vi "count from data base_0.vi"() -> ()   [LabVIEW 2015]
panel:
  in  "Tab Control":enum32{"Page 1", "Page 2"}(tab)
  out "Array":dbl[](array[numeric])
  in  "?":dbl
  out "Result":i16
  # "Count from data base"
  # "User enter value__ count in result how much int value greater than user enput"
  # "Pardeep Kumar"
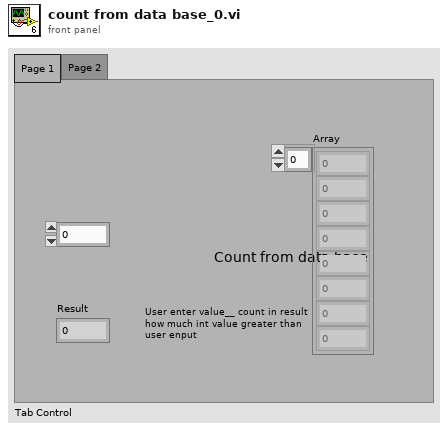
[diagram p1: front panel]
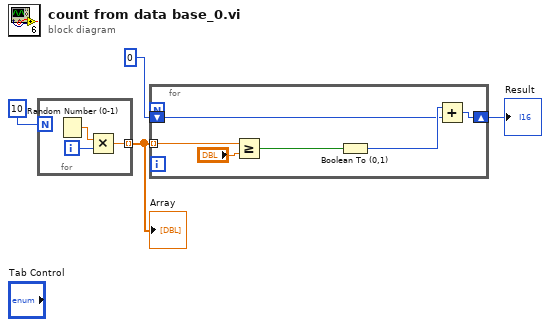
[diagram p0: block diagram]
diagram:
  n1 = for {
    N: 10 -> [_]
    tunnel: [w5] -> w3 mode=indexing
    i -> [w6]
    n2 = Random Number (0-1)() -> (number: 0 to 1=w7:dbl)
    n3 = Multiply(x=w7, y=w6) -> (x*y=w5:dbl)
  }
  "Array" <- w3
  n4 = for {
    tunnel: w3 -> [w13] mode=indexing
    shift-right: [w9] -> w2
    shift-left: i16 0 -> [w8]
    n5 = Greater Or Equal?(x=w13, y="?") -> (x >= y?=w11:bool)
    n6 = Boolean To (0,1)(Boolean=w11) -> (0, 1=w10:i16)
    n7 = Add(x=w10, y=w8) -> (x+y=w9:i16)
  }
  "Result" <- w2
